vi "SDSU.vi"(8 "error in":errorcluster, 9 "arguments":string, 10 "function":string, 11 "fd in":i32) -> (0 "error out":errorcluster, 1 "result type":string, 2 "str result":string, 3 "fd out":i32)   [LabVIEW 2016]
uses:
  DBSHAND/private/vis/DatabaseHand_Element_Get(bool).vi
  DBSHAND/private/vis/DatabaseHand_Element_Set(bool).vi
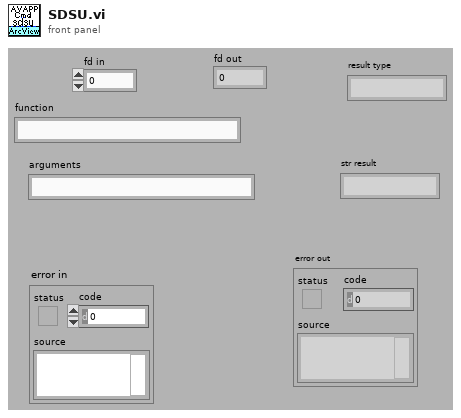
[diagram p1: front panel]
types:
  T1 = cluster{"Video Processor Type":string, "support gain":bool, "Timing Board":string, "support reset":bool, "Utility Board":string, "Shutter":string, "Temperature":string, "support temp control":bool, "Detector Type":string, "Support MPP":string, "Support Binning":string, "Readout Mode":string, "support shutter control":bool}
  T2 = typedef "DatabaseHand_RefNum.ctl" = refnum<vi>
  T3 = typedef "CMN_ContStatus.ctl" = cluster{"Response":string, "power":bool, "shutter":bool, "artifdata":bool, "idlemode":bool, "reset":bool, "gain":u8, "speed":u8, "resetPCI":bool, "autoshutter":bool, "TempSetPoint":i32, "multipleextensions":bool, "displayImage":bool, "coadding":bool, "images being coadded":i32, "Operation Mode":enum16{"normal", "coadd", "fawler"}, "frames to write":cluster{"subs":bool, "reset":bool, "exposed":bool}, "fawler samples":i32, "write auto":bool, "datatype":string, "frames to display":cluster{"subs":bool, "reset":bool, "exposed":bool}, "sur":i32, "autoclear":bool}
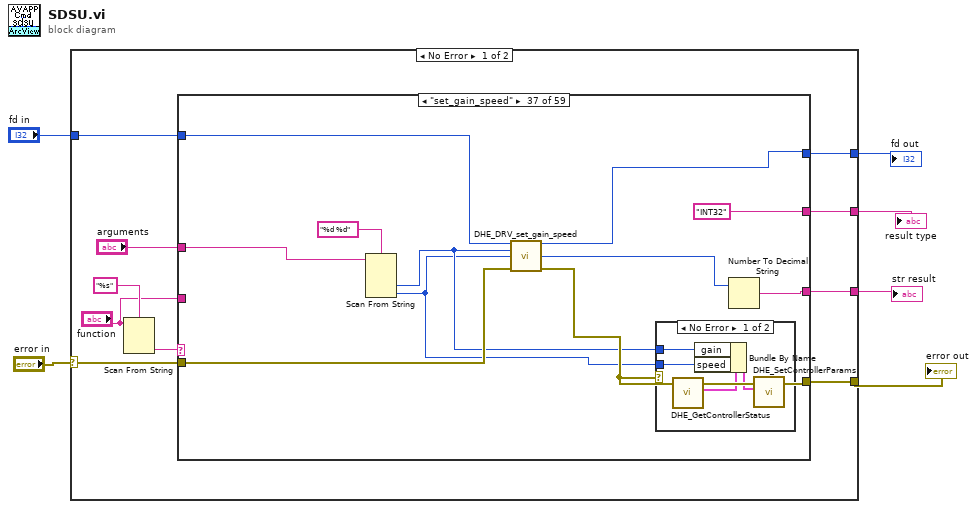
[diagram p0: block diagram]
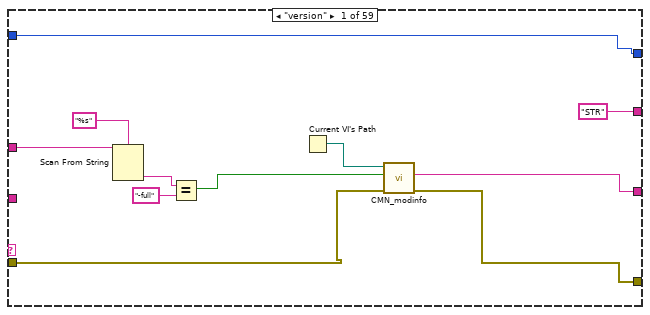
[diagram p2: hidden frame]
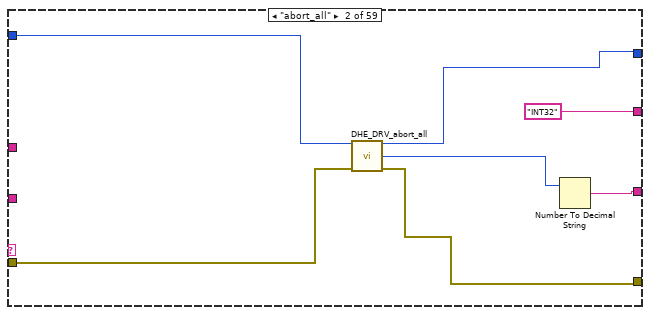
[diagram p3: hidden frame]
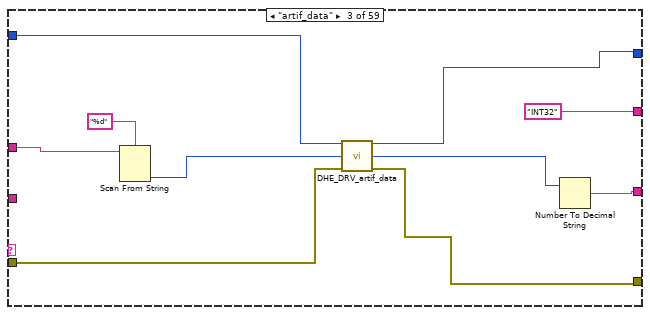
[diagram p4: hidden frame]
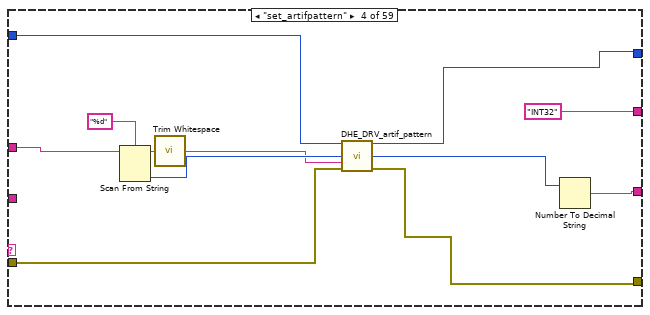
[diagram p5: hidden frame]
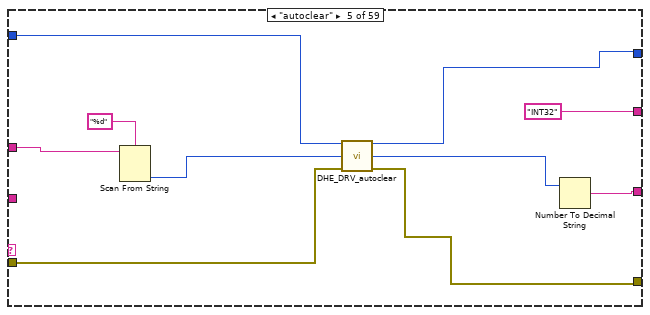
[diagram p6: hidden frame]
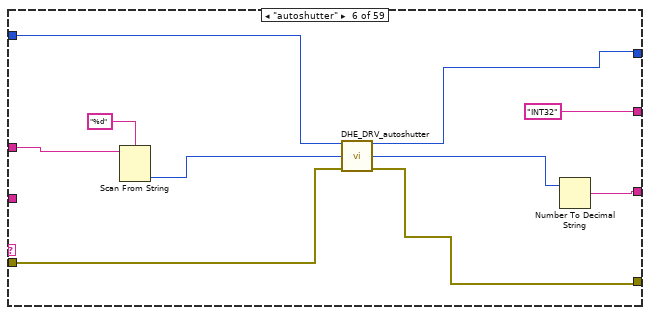
[diagram p7: hidden frame]
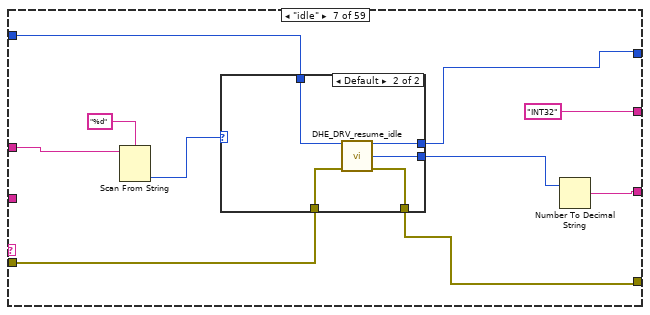
[diagram p8: hidden frame]
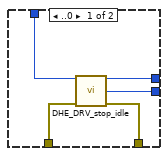
[diagram p9: hidden frame]
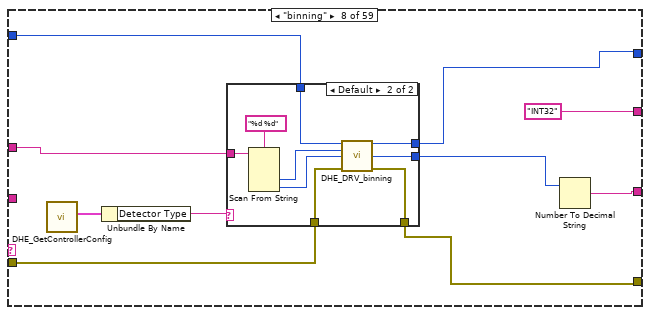
[diagram p10: hidden frame]
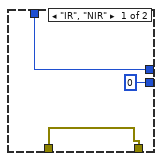
[diagram p11: hidden frame]
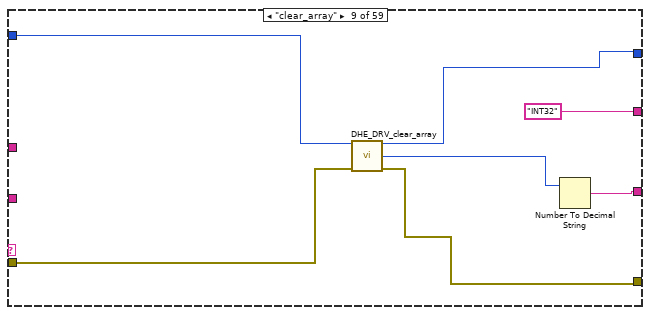
[diagram p12: hidden frame]
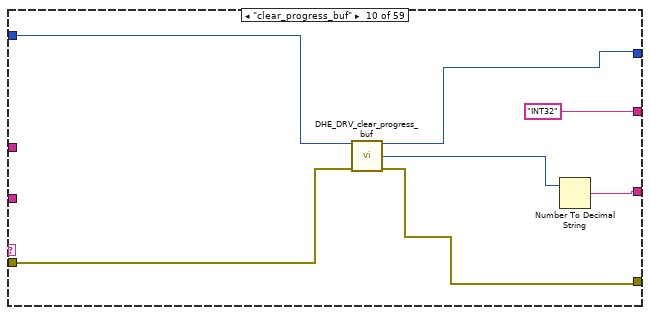
[diagram p13: hidden frame]
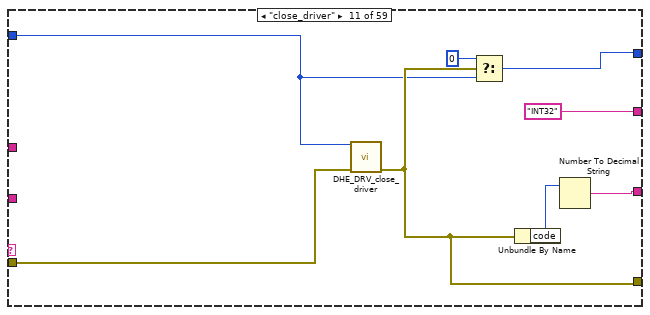
[diagram p14: hidden frame]
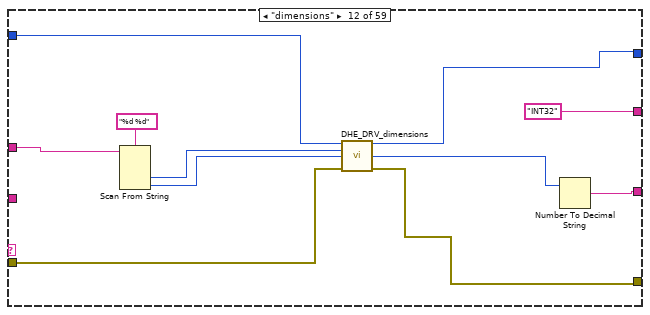
[diagram p15: hidden frame]
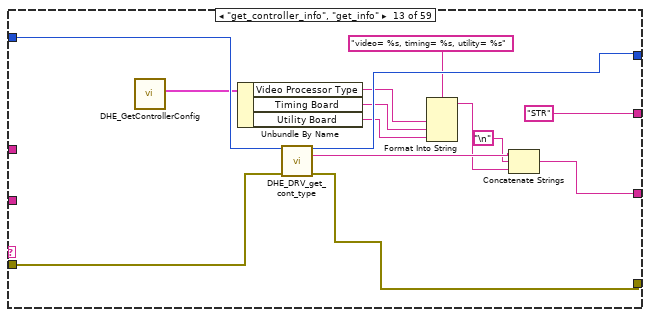
[diagram p16: hidden frame]
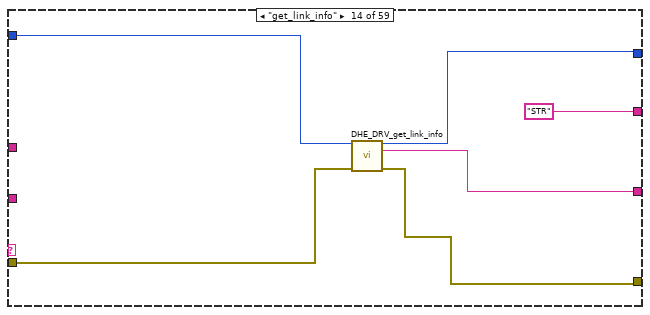
[diagram p17: hidden frame]
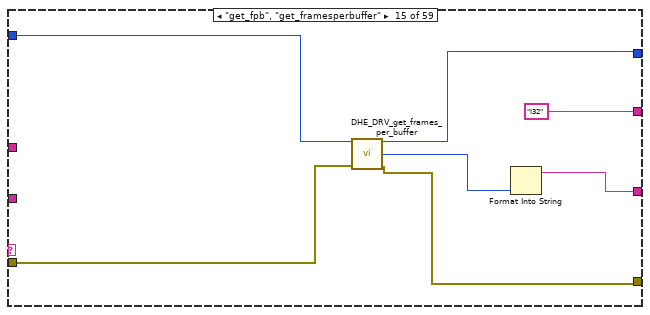
[diagram p18: hidden frame]
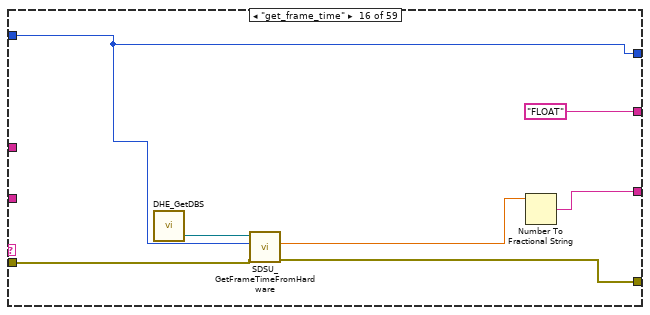
[diagram p19: hidden frame]
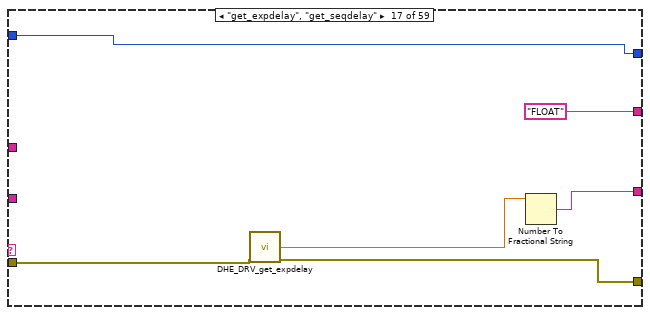
[diagram p20: hidden frame]
diagram:
  n1 = case shown="No Error" "error in" {
    selector: "error in" -> [w10 w645]
    tunnel: [w11 w645] -> w6
    tunnel: [w15 w644] -> w4
    tunnel: "fd in" -> [w14 w644]
    tunnel: [w13 w643] -> w2
    tunnel: [w12 w643] -> w1
    frame No Error {
      n2 = Scan From String(format string="%s", input string="function") -> (output 1=w8:string)  [unwired: 2 in, 4 out]
      n3 = case shown="\"set_gain_speed\"" w8 {
        tunnel: w10 -> [w18 w31 w42 w54 w64 w74 w84 w104 w122 w129 w139 w149 w163 w170 w174 w181 w188 w194 w202 w211 w221 w226 w236 w240 w250 w261 w272 w287 w294 w301 w312 w322 w333 w339 w346 w358 w369 w383 w394 w409 w420 w429 w435 w442 w452 w461 w470 w476 w488 w510 w539 w554 w587 w593 w600 w609 w619 w625 w639]
        tunnel: "arguments" -> [w23 _ w37 w49 w59 w69 w79 w99 _ _ _ w144 _ _ _ _ _ _ _ _ _ _ w231 w246 _ w256 w270 w283 _ _ w307 w317 w329 _ _ w354 w366 w378 w389 w404 w415 w426 _ _ w454 w463 w472 w484 w496 w511 w535 w553 w582 _ _ w605 w621 w629 w636]
        tunnel: [w24 w28 w39 w51 w61 w71 w81 w101 w119 w126 w134 w146 w161 w167 w176 w182 w189 w195 w203 w212 w222 w228 w233 w243 w247 w258 w274 w289 w291 w298 w309 w319 w331 w336 w344 w356 w368 w380 w391 w406 w417 w424 w432 w439 w449 w459 w468 w479 w493 w509 w536 w556 w584 w590 w599 w606 w615 w626 w640] -> w15
        tunnel: w14 -> [w24 w32 w40 w52 w62 w72 w82 w102 w123 w130 w135 w147 w164 w168 w177 w182 w189 w195 w203 w212 w222 w228 w234 _ w251 w259 w275 w290 w295 w302 w310 w320 w327 w340 w347 w352 w364 w381 w392 w407 w418 w424 w432 w440 w450 w459 w468 w480 w494 w509 w540 w557 w585 w594 w599 w607 w616 w627 w641]
        tunnel: [w26 w33 w43 w55 w65 w75 w85 w105 w124 w131 w137 w150 w152 w166 w173 w184 w190 w196 w204 w207 w216 w223 w237 w242 w252 w262 w271 w286 w296 w303 w313 w323 w334 w341 w348 w359 w370 w384 w395 w410 w421 w430 w436 w443 w455 w464 w473 w485 w497 w512 w541 w544 w588 w595 w601 w604 w617 w623 w637] -> w13
        tunnel: ["STR" "INT32" "INT32" "INT32" "INT32" "INT32" "INT32" "INT32" "INT32" "INT32" "INT32" "INT32" "STR" "STR" "I32" "FLOAT" "FLOAT" "FLOAT" "FLOAT" "STR" "STR" "STR" "INT32" "INT32" "INT32" "INT32" "STR" "STR" "INT32" "INT32" "INT32" "INT32" "INT32" "INT32" "INT32" "INT32" "INT32" "INT32" "INT32" "INT32" "INT32" "INT32" "INT32" "FLOAT" "INT32" "INT32" "INT32" "INT32" "INT32" "INT32" "INT32" "INT32" "INT32" "INT32" "INT32" "STR" "STR" "STR" "STR"] -> w12
        tunnel: [w17 w30 w41 w53 w63 w73 w83 w103 w121 w128 w136 w148 w162 w169 w175 w180 w187 w193 w201 w211 w221 w225 w235 w239 w249 w260 w273 w288 w293 w300 w311 w321 w332 w338 w345 w357 w363 w382 w393 w408 w419 w428 w434 w441 w451 w460 w469 w475 w487 w503 w538 w555 w586 w592 w598 w608 w618 w624 w638] -> w11
        tunnel: "function" -> [_ _ _ _ _ _ _ _ _ _ _ _ _ _ _ _ _ _ _ _ _ _ _ _ _ _ _ _ _ _ _ _ _ _ _ _ _ _ _ _ _ _ _ _ _ _ _ _ _ _ _ _ _ _ _ _ _ w631 _]
        frame "version" {
          n4 = Scan From String(format string="%s", input string=w23) -> (output 1=w21:string)  [unwired: 2 in, 4 out]
          n5 = Equal?(x=w21, y="-full") -> (x = y?=w19:bool)
          n6 = Current VI's Path() -> (path=w27:path)
          n7 = call "CMN_modinfo.vi"("error in (no error)"=w18, "full"=w19, "caller path"=w27) -> ("error out"=w17:errorcluster, "INFO"=w26:string)  [unwired: 7 out]
        }
        frame "abort_all" {
          n8 = call "DHE_DRV_abort_all.vi"("fd"=w32, "error in (no error)"=w31) -> ("fd out"=w28:i32, "return value"=w29:i32, "error out"=w30:errorcluster)  [unwired: 11 out]
          n9 = Number To Decimal String(number=w29) -> (decimal integer string=w33:string)  [unwired: 1 out]
        }
        frame "artif_data" {
          n10 = Scan From String(format string="%d", input string=w37) -> (output 1=w35:i32)  [unwired: 2 in, 4 out]
          n11 = call "DHE_DRV_artif_data.vi"("fd"=w40, "flag"=w35, "error in (no error)"=w42) -> ("fd out"=w39:i32, "return value"=w38:i32, "error out"=w41:errorcluster)  [unwired: 10 out]
          n12 = Number To Decimal String(number=w38) -> (decimal integer string=w43:string)  [unwired: 1 out]
        }
        frame "set_artifpattern" {
          n13 = Scan From String(format string="%d", input string=w49) -> (remaining string=w46:string, output 1=w47:i32)  [unwired: 2 in, 3 out]
          n14 = call <vilib>:"Trim Whitespace.vi"("string"=w46) -> ("trimmed string"=w45:string)  [unwired: 1 in]
          n15 = call "DHE_DRV_artif_pattern.vi"("fd"=w52, "type"=w47, "params"=w45, "error in (no error)"=w54) -> ("fd out"=w51:i32, "return value"=w50:i32, "error out"=w53:errorcluster)  [unwired: 9 out]
          n16 = Number To Decimal String(number=w50) -> (decimal integer string=w55:string)  [unwired: 1 out]
        }
        frame "autoclear" {
          n17 = Scan From String(format string="%d", input string=w59) -> (output 1=w57:i32)  [unwired: 2 in, 4 out]
          n18 = call "DHE_DRV_autoclear.vi"("fd"=w62, "flag"=w57, "error in (no error)"=w64) -> ("fd out"=w61:i32, "return value"=w60:i32, "error out"=w63:errorcluster)  [unwired: 10 out]
          n19 = Number To Decimal String(number=w60) -> (decimal integer string=w65:string)  [unwired: 1 out]
        }
        frame "autoshutter" {
          n20 = Scan From String(format string="%d", input string=w69) -> (output 1=w67:i32)  [unwired: 2 in, 4 out]
          n21 = call "DHE_DRV_autoshutter.vi"("fd"=w72, "flag"=w67, "error in (no error)"=w74) -> ("fd out"=w71:i32, "return value"=w70:i32, "error out"=w73:errorcluster)  [unwired: 10 out]
          n22 = Number To Decimal String(number=w70) -> (decimal integer string=w75:string)  [unwired: 1 out]
        }
        frame "idle" {
          n23 = Scan From String(format string="%d", input string=w79) -> (output 1=w77:i32)  [unwired: 2 in, 4 out]
          n24 = case shown="Default" w77 {
            tunnel: w84 -> [w91 w96]
            tunnel: [w90 w95] -> w83
            tunnel: w82 -> [w89 w94]
            tunnel: [w88 w93] -> w81
            tunnel: [w87 w92] -> w80
            frame ..0 {
              n25 = call "DHE_DRV_stop_idle.vi"("fd"=w89, "error in (no error)"=w91) -> ("fd out"=w88:i32, "return value"=w87:i32, "error out"=w90:errorcluster)  [unwired: 11 out]
            }
            frame Default {
              n26 = call "DHE_DRV_resume_idle.vi"("fd"=w94, "error in (no error)"=w96) -> ("fd out"=w93:i32, "return value"=w92:i32, "error out"=w95:errorcluster)  [unwired: 11 out]
            }
          }
          n27 = Number To Decimal String(number=w80) -> (decimal integer string=w85:string)  [unwired: 1 out]
        }
        frame "binning" {
          n28 = call "DHE_GetControllerConfig.vi"() -> ("ControllerConfigCluster"=w98:T1)  [unwired: 11 out]
          n29 = Unbundle By Name(w98) -> ("Detector Type"=w97:string)
          n30 = case shown="Default" w97 {
            tunnel: w104 -> [w107 w118]
            tunnel: [w107 w117] -> w103
            tunnel: w102 -> [w109 w116]
            tunnel: [w109 w115] -> w101
            tunnel: [0 ("return value") w114] -> w100
            tunnel: w99 -> [_ w113]
            frame "IR", "NIR" {
            }
            frame Default {
              n31 = Scan From String(format string="%d %d", input string=w113) -> (output 1=w111:i32, output 2=w110:i32)  [unwired: 2 in, 5 out]
              n32 = call "DHE_DRV_binning.vi"("fd"=w116, "xbin"=w111, "ybin"=w110, "error in (no error)"=w118) -> ("fd out"=w115:i32, "return value"=w114:i32, "error out"=w117:errorcluster)  [unwired: 9 out]
            }
          }
          n33 = Number To Decimal String(number=w100) -> (decimal integer string=w105:string)  [unwired: 1 out]
        }
        frame "clear_array" {
          n34 = call "DHE_DRV_clear_array.vi"("fd"=w123, "error in (no error)"=w122) -> ("fd out"=w119:i32, "return value"=w120:i32, "error out"=w121:errorcluster)  [unwired: 11 out]
          n35 = Number To Decimal String(number=w120) -> (decimal integer string=w124:string)  [unwired: 1 out]
        }
        frame "clear_progress_buf" {
          n36 = call "DHE_DRV_clear_progress_buf.vi"("fd"=w130, "error in (no error)"=w129) -> ("fd"=w126:i32, "return value"=w127:i32, "error out"=w128:errorcluster)  [unwired: 11 out]
          n37 = Number To Decimal String(number=w127) -> (decimal integer string=w131:string)  [unwired: 1 out]
        }
        frame "close_driver" {
          n38 = call "DHE_DRV_close_driver.vi"("fd"=w135, "error in (no error)"=w139) -> ("error out"=w136:errorcluster)  [unwired: 13 out]
          n39 = Select(t=0, s=w136, f=w135) -> (s? t:f=w134:i32)
          n40 = Unbundle By Name(w136) -> ("code"=w138:i32)
          n41 = Number To Decimal String(number=w138) -> (decimal integer string=w137:string)  [unwired: 1 out]
        }
        frame "dimensions" {
          n42 = Scan From String(format string="%d %d", input string=w144) -> (output 1=w142:i32, output 2=w141:i32)  [unwired: 2 in, 5 out]
          n43 = call "DHE_DRV_dimensions.vi"("fd"=w147, "Columns"=w142, "Rows"=w141, "error in (no error)"=w149) -> ("fd out"=w146:i32, "return value"=w145:i32, "error out"=w148:errorcluster)  [unwired: 9 out]
          n44 = Number To Decimal String(number=w145) -> (decimal integer string=w150:string)  [unwired: 1 out]
        }
        frame "get_controller_info", "get_info" {
          n45 = call "DHE_GetControllerConfig.vi"() -> ("ControllerConfigCluster"=w160:T1)  [unwired: 11 out]
          n46 = Unbundle By Name(w160) -> ("Video Processor Type"=w157:string, "Timing Board"=w156:string, "Utility Board"=w155:string)
          n47 = call "DHE_DRV_get_cont_type.vi"("fd"=w164, "error in (no error)"=w163) -> ("fd out"=w161:i32, "info out"=w159:string, "error out"=w162:errorcluster)  [unwired: 11 out]
          n48 = Format Into String(format string="video= %s, timing= %s, utility= %s", w157, w156, w155) -> (resulting string=w153:string)  [unwired: 2 in, 1 out]
          n49 = Concatenate Strings(w159, "\n", w153) -> (w152:string)
        }
        frame "get_link_info" {
          n50 = call "DHE_DRV_get_link_info.vi"("fd"=w168, "error in (no error)"=w170) -> ("fd out"=w167:i32, "info out"=w166:string, "error out"=w169:errorcluster)  [unwired: 11 out]
        }
        frame "get_fpb", "get_framesperbuffer" {
          n51 = call "DHE_DRV_get_frames_per_buffer.vi"("fd"=w177, "error in (no error)"=w174) -> ("fd"=w176:i32, "fpb"=w172:i32, "error out"=w175:errorcluster)  [unwired: 11 out]
          n52 = Format Into String(w172) -> (resulting string=w173:string)  [unwired: 3 in, 1 out]
        }
        frame "get_frame_time" {
          n53 = call "DHE_GetDBS.vi"() -> ("DHE_DBSRef"=w183:T2)  [unwired: 9 out]
          n54 = call "SDSU_GetFrameTimeFromHardware.vi"("error in"=w181, "fd"=w182, "Database Ref"=w183) -> ("errorout"=w180:errorcluster, "frame_time"=w179:dbl)  [unwired: 7 out]
          n55 = Number To Fractional String(number=w179) -> (F-format string=w184:string)  [unwired: 3 out]
        }
        frame "get_expdelay", "get_seqdelay" {
          n56 = call "DHE_DRV_get_expdelay.vi"("error in (no error)"=w188) -> ("delay"=w186:sgl, "error out"=w187:errorcluster)  [unwired: 2 in, 11 out]
          n57 = Number To Fractional String(number=w186) -> (F-format string=w190:string)  [unwired: 3 out]
        }
        frame "get_iniexpdelay", "get_iniseqdelay", "get_initdelay", "get_intdelay" {
          n58 = call "DHE_DRV_get_iniexpdelay.vi"("error in (no error)"=w194) -> ("delay"=w192:sgl, "error out"=w193:errorcluster)  [unwired: 13 out]
          n59 = Number To Fractional String(number=w192) -> (F-format string=w196:string)  [unwired: 3 out]
        }
        frame "get_act_inttime", "get_actual_inttime", "get_hard_inttime" {
          n60 = call "DHE_DRV_get_actual_inttime.vi"("error in (no error)"=w202) -> ("actual inttime"=w200:i32, "error out"=w201:errorcluster)  [unwired: 13 out]
          n61 = Divide(x=w200, y=1000) -> (x/y=w198:dbl)
          n62 = Number To Fractional String(number=w198) -> (F-format string=w204:string)  [unwired: 3 out]
        }
        frame "get_samplings" {
          n63 = call "DHE_GetControllerConfig.vi"() -> ("ControllerConfigCluster"=w210:T1)  [unwired: 11 out]
          n64 = Unbundle By Name(w210) -> ("Detector Type"=w209:string)
          n65 = To Lower Case(string=w209) -> (all lower case string=w208:string)
          n66 = case shown="Default" w208 {
            tunnel: ["single, singframe" "single, cds, fowler, sur"] -> w207
            frame Default {
            }
            frame "ir", "nir" {
            }
          }
        }
        frame "get_sync" {
          n67 = call "DHE_GetDBS.vi"() -> ("DHE_DBSRef"=w215:T2)  [unwired: 9 out]
          n68 = call-poly "DatabaseHand_Get.vi"("default value"=FALSE, "name"="synced", "Database RefNum in"=w215) -> ("value"=w217:bool)  [unwired: 2 in, 6 out]
          n69 = Format Into String(w217) -> (resulting string=w216:string)  [unwired: 3 in, 1 out]
        }
        frame "get_guide_mode" {
          n70 = call "DHE_DRV_get_guide_mode.vi"("error in (no error)"=w226) -> ("guide_mode"=w224:bool, "error out"=w225:errorcluster)  [unwired: 13 out]
          n71 = Format Into String(w224) -> (resulting string=w223:string)  [unwired: 3 in, 1 out]
        }
        frame "move_shutter" {
          n72 = Scan From String(format string="%d", input string=w231) -> (output 1=w229:i32)  [unwired: 2 in, 4 out]
          n73 = call "DHE_DRV_move_shutter.vi"("fd"=w234, "flag"=w229, "error in (no error)"=w236) -> ("fd out"=w233:i32, "return value"=w232:i32, "error out"=w235:errorcluster)  [unwired: 10 out]
          n74 = Number To Decimal String(number=w232) -> (decimal integer string=w237:string)  [unwired: 1 out]
        }
        frame "open_driver" {
          n75 = Scan From String(format string="%d", input string=w246) -> (output 1=w244:i32)  [unwired: 2 in, 4 out]
          n76 = call "DHE_DRV_open_driver.vi"("devno"=w244, "error in (no error)"=w240) -> ("refnum"=w243:i32, "error out"=w239:errorcluster)  [unwired: 12 out]
          n77 = Format Into String(w243) -> (resulting string=w242:string)  [unwired: 3 in, 1 out]
        }
        frame "pause_exposure" {
          n78 = call "DHE_DRV_pause_exposure.vi"("fd"=w251, "error in (no error)"=w250) -> ("fd out"=w247:i32, "return value"=w248:i32, "error out"=w249:errorcluster)  [unwired: 11 out]
          n79 = Number To Decimal String(number=w248) -> (decimal integer string=w252:string)  [unwired: 1 out]
        }
        frame "power" {
          n80 = Scan From String(format string="%d", input string=w256) -> (output 1=w254:i32)  [unwired: 2 in, 4 out]
          n81 = call "DHE_DRV_power.vi"("fd"=w259, "flag"=w254, "error in (no error)"=w261) -> ("fd out"=w258:i32, "return value"=w257:i32, "error out"=w260:errorcluster)  [unwired: 10 out]
          n82 = Number To Decimal String(number=w257) -> (decimal integer string=w262:string)  [unwired: 1 out]
        }
        frame "read_memory", "read_temperature", "read_tp" {
          # "board memory address"
          n83 = Scan From String(format string="%s %s %s", input string=w270) -> (output 1=w268:string, output 2=w267:string, output 3=w266:string)  [unwired: 2 in, 6 out]
          n84 = Format Into String(format string="read %s %s %s " ("string"), w268, w267, w266) -> (resulting string=w265:string)  [unwired: 2 in, 1 out]
          n85 = call "SDSU_Memory.vi"("refnum"=w275, "Command In"=w265, "error in (no error)"=w272) -> ("refnum out"=w274:i32, "message"=w271:string, "error out"=w273:errorcluster)  [unwired: 2 in, 8 out]
        }
        frame "write_memory", "write_tp" {
          # "board memory address type value name"
          # "board memory address value"
          n86 = Scan From String(format string="%s %s %s %s %s %s ", input string=w283) -> (output 1=w284:string, output 2=w282:string, output 3=w281:string, output 5=w279:string)  [unwired: 2 in, 11 out]
          n87 = Format Into String(format string="write %s %s %s %s " ("string"), w284, w282, w281, w279) -> (resulting string=w277:string)  [unwired: 2 in, 1 out]
          n88 = call "SDSU_Memory.vi"("refnum"=w290, "Command In"=w277, "error in (no error)"=w287) -> ("refnum out"=w289:i32, "message"=w286:string, "error out"=w288:errorcluster)  [unwired: 2 in, 8 out]
        }
        frame "reset_controller" {
          n89 = call "DRV_SDSU_reset_ctrler.vi"("fd"=w295, "error in (no error)"=w294) -> ("fd out"=w291:i32, "return value"=w292:i32, "error out"=w293:errorcluster)  [unwired: 11 out]
          n90 = Number To Decimal String(number=w292) -> (decimal integer string=w296:string)  [unwired: 1 out]
        }
        frame "resume_exposure" {
          n91 = call "DHE_DRV_resume_exposure.vi"("fd"=w302, "error in (no error)"=w301) -> ("fd out"=w298:i32, "return value"=w299:i32, "error out"=w300:errorcluster)  [unwired: 11 out]
          n92 = Number To Decimal String(number=w299) -> (decimal integer string=w303:string)  [unwired: 1 out]
        }
        frame "set_bpp" {
          n93 = Scan From String(format string="%d", input string=w307) -> (output 1=w305:i32)  [unwired: 2 in, 4 out]
          n94 = call "DHE_DRV_set_bpp.vi"("fd"=w310, "bpp"=w305, "error in (no error)"=w312) -> ("fd out"=w309:i32, "return value"=w308:i32, "error out"=w311:errorcluster)  [unwired: 10 out]
          n95 = Number To Decimal String(number=w308) -> (decimal integer string=w313:string)  [unwired: 1 out]
        }
        frame "set_pixel_time", "set_pixeltime", "set_pixtime" {
          n96 = Scan From String(format string="%g", input string=w317) -> (output 1=w315:dbl)  [unwired: 2 in, 4 out]
          n97 = call "DHE_DRV_set_pixeltime.vi"("fd"=w320, "pixtime"=w315, "error in (no error)"=w322) -> ("fd out"=w319:i32, "return value"=w318:i32, "error out"=w321:errorcluster)  [unwired: 10 out]
          n98 = Number To Decimal String(number=w318) -> (decimal integer string=w323:string)  [unwired: 1 out]
        }
        frame "set_gain" {
          n99 = call "DHE_DRV_get_gain_speed.vi"("fd"=w327) -> ("speed"=w325:i32)  [unwired: 10 in, 4 out]
          n100 = Scan From String(format string="%d", input string=w329) -> (output 1=w326:i32)  [unwired: 2 in, 4 out]
          n101 = call "DHE_DRV_set_gain_speed.vi"("fd"=w327, "gain"=w326, "speed"=w325, "error in (no error)"=w333) -> ("fd out"=w331:i32, "return value"=w330:i32, "error out"=w332:errorcluster)  [unwired: 9 in]
          n102 = Number To Decimal String(number=w330) -> (decimal integer string=w334:string)  [unwired: 1 out]
        }
        frame "get_gain" {
          n103 = call "DHE_DRV_get_gain_speed.vi"("fd"=w340, "error in (no error)"=w339) -> ("fd out"=w336:i32, "gain"=w337:i32, "error out"=w338:errorcluster)  [unwired: 9 in, 2 out]
          n104 = Number To Decimal String(number=w337) -> (decimal integer string=w341:string)  [unwired: 1 out]
        }
        frame "get_speed" {
          n105 = call "DHE_DRV_get_gain_speed.vi"("fd"=w347, "error in (no error)"=w346) -> ("fd out"=w344:i32, "speed"=w343:i32, "error out"=w345:errorcluster)  [unwired: 9 in, 2 out]
          n106 = Number To Decimal String(number=w343) -> (decimal integer string=w348:string)  [unwired: 1 out]
        }
        frame "set_speed" {
          n107 = call "DHE_DRV_get_gain_speed.vi"("fd"=w352) -> ("gain"=w351:i32)  [unwired: 10 in, 4 out]
          n108 = Scan From String(format string="%d", input string=w354) -> (output 1=w350:i32)  [unwired: 2 in, 4 out]
          n109 = call "DHE_DRV_set_gain_speed.vi"("fd"=w352, "gain"=w351, "speed"=w350, "error in (no error)"=w358) -> ("fd out"=w356:i32, "return value"=w355:i32, "error out"=w357:errorcluster)  [unwired: 9 in]
          n110 = Number To Decimal String(number=w355) -> (decimal integer string=w359:string)  [unwired: 1 out]
        }
        frame "set_gain_speed" {
          n111 = Scan From String(format string="%d %d", input string=w366) -> (output 1=w362:i32, output 2=w361:i32)  [unwired: 2 in, 5 out]
          n112 = call "DHE_DRV_set_gain_speed.vi"("fd"=w364, "gain"=w362, "speed"=w361, "error in (no error)"=w369) -> ("fd out"=w368:i32, "return value"=w367:i32, "error out"=w363:errorcluster)  [unwired: 9 in]
          n113 = case shown="No Error" w363 {
            tunnel: w362 -> [w373 _]
            tunnel: w361 -> [w372 _]
            frame No Error {
              n114 = call "DHE_GetControllerStatus.vi"() -> ("ControllerStatus"=w375:T3)  [unwired: 11 out]
              n115 = Bundle By Name(cluster=w375, "gain"=w373, "speed"=w372) -> (w374:T3)
              n116 = call "DHE_SetControllerParams.vi"("ControllerStatus"=w374) -> ()  [unwired: 1 in, 10 out]
            }
            frame Error {
            }
          }
          n117 = Number To Decimal String(number=w367) -> (decimal integer string=w370:string)  [unwired: 1 out]
        }
        frame "framesperbuffer", "set_fpb", "set_framesperbuffer" {
          n118 = Scan From String(format string="%d", input string=w378) -> (output 1=w376:i32)  [unwired: 2 in, 4 out]
          n119 = call "DHE_DRV_set_fpb.vi"("fd"=w381, "fpb"=w376, "error in (no error)"=w383) -> ("fd out"=w380:i32, "return value"=w379:i32, "error out"=w382:errorcluster)  [unwired: 10 out]
          n120 = Number To Decimal String(number=w379) -> (decimal integer string=w384:string)  [unwired: 1 out]
        }
        frame "set_exp_time" {
          n121 = Scan From String(format string="%d", input string=w389) -> (output 1=w387:i32)  [unwired: 2 in, 4 out]
          n122 = To Unsigned Long Integer(number=w387) -> (unsigned 32bit integer=w386:u32)
          n123 = call "DHE_DRV_set_exp_time.vi"("fd"=w392, "val"=w386, "error in (no error)"=w394) -> ("fd out"=w391:i32, "return value"=w390:i32, "error out"=w393:errorcluster)  [unwired: 10 out]
          n124 = Number To Decimal String(number=w390) -> (decimal integer string=w395:string)  [unwired: 1 out]
        }
        frame "set_geom" {
          # "xpre xdata xpost ypre ydata ypost"
          n125 = Scan From String(format string="%d %d %d %d %d %d", input string=w404) -> (output 1=w402:i32, output 2=w401:i32, output 3=w400:i32, output 4=w398:i32, output 5=w399:i32, output 6=w397:i32)  [unwired: 2 in, 9 out]
          n126 = call "DHE_DRV_set_geom.vi"("fd"=w407, "ypredata"=w398, "ypostdata"=w397, "xpredata"=w402, "xpostdata"=w400, "xdata"=w401, "error in (no error)"=w409, "ydata"=w399) -> ("fd out"=w406:i32, "return value"=w405:i32, "error out"=w408:errorcluster)  [unwired: 5 out]
          n127 = Number To Decimal String(number=w405) -> (decimal integer string=w410:string)  [unwired: 1 out]
        }
        frame "set_nimages" {
          n128 = Scan From String(format string="%d", input string=w415) -> (output 1=w413:i32)  [unwired: 2 in, 4 out]
          n129 = To Unsigned Long Integer(number=w413) -> (unsigned 32bit integer=w412:u32)
          n130 = call "DHE_DRV_set_nimages.vi"("fd"=w418, "nimages"=w412, "error in (no error)"=w420) -> ("fd out"=w417:i32, "return value"=w416:i32, "error out"=w419:errorcluster)  [unwired: 10 out]
          n131 = Number To Decimal String(number=w416) -> (decimal integer string=w421:string)  [unwired: 1 out]
        }
        frame "set_mapping", "set_mapsize" {
          n132 = Scan From String(format string="%d", input string=w426) -> (output 1=w423:i32)  [unwired: 2 in, 4 out]
          n133 = call "DHE_DRV_set_mapsize.vi"("size_MB"=w423, "error in (no error)"=w429) -> ("return value"=w427:i32, "error out"=w428:errorcluster)  [unwired: 2 in, 10 out]
          n134 = Number To Decimal String(number=w427) -> (decimal integer string=w430:string)  [unwired: 1 out]
        }
        frame "get_mapping", "get_mapsize" {
          n135 = call "DHE_DRV_get_mapsize.vi"("error in (no error)"=w435) -> ("return value"=w433:i32, "error out"=w434:errorcluster)  [unwired: 1 in, 12 out]
          n136 = Number To Decimal String(number=w433) -> (decimal integer string=w436:string)  [unwired: 1 out]
        }
        frame "get_pixel_time", "get_pixeltime", "get_pixtime" {
          n137 = call "DHE_DRV_get_pixtime.vi"("fd"=w440, "error in (no error)"=w442) -> ("fd out"=w439:i32, "pixtime"=w438:sgl, "error out"=w441:errorcluster)  [unwired: 11 out]
          n138 = Number To Fractional String(number=w438) -> (F-format string=w443:string)  [unwired: 3 out]
        }
        frame "set_nsur" {
          n139 = Scan From String(format string="%d", input string=w454) -> (output 1=w446:i32)  [unwired: 2 in, 4 out]
          n140 = Max & Min(x=w446, y=1) -> (max(x,y)=w445:i32)  [unwired: 1 out]
          n141 = call "DHE_DRV_set_num_sur.vi"("fd"=w450, "num_reads"=w445, "error in (no error)"=w452) -> ("fd out"=w449:i32, "return value"=w448:i32, "error out"=w451:errorcluster)  [unwired: 10 out]
          n142 = Number To Decimal String(number=w448) -> (decimal integer string=w455:string)  [unwired: 1 out]
        }
        frame "set_expdelay", "set_seqdelay" {
          n143 = Scan From String(format string="%g", input string=w463) -> (output 1=w458:dbl)  [unwired: 2 in, 4 out]
          n144 = call "DHE_DRV_set_expdelay.vi"("delay(ms)"=w458, "error in (no error)"=w461) -> ("error out"=w460:errorcluster)  [unwired: 1 in, 12 out]
          n145 = Number To Decimal String(number=0) -> (decimal integer string=w464:string)  [unwired: 1 out]
        }
        frame "set_inidelay", "set_iniexpdelay", "set_iniseqdelay", "set_intdelay" {
          n146 = Scan From String(format string="%g", input string=w472) -> (output 1=w466:dbl)  [unwired: 2 in, 4 out]
          n147 = call "DHE_DRV_set_iniexpdelay.vi"("delay(ms)"=w466, "error in (no error)"=w470) -> ("error out"=w469:errorcluster)  [unwired: 1 in, 12 out]
          n148 = Number To Decimal String(number=0) -> (decimal integer string=w473:string)  [unwired: 1 out]
        }
        frame "set_ncoadds" {
          n149 = Scan From String(format string="%d", input string=w484) -> (output 1=w481:i32)  [unwired: 2 in, 4 out]
          n150 = Max & Min(x=w481, y=1) -> (max(x,y)=w478:i32)  [unwired: 1 out]
          n151 = call "DHE_DRV_set_num_coadds.vi"("fd"=w480, "num_coadds"=w478, "error in (no error)"=w476) -> ("fd out"=w479:i32, "return value"=w477:i32, "error out"=w475:errorcluster)  [unwired: 10 out]
          n152 = Number To Decimal String(number=w477) -> (decimal integer string=w485:string)  [unwired: 1 out]
        }
        frame "set_fowler", "set_fsamples" {
          n153 = Scan From String(format string="%d", input string=w496) -> (output 1=w491:i32)  [unwired: 2 in, 4 out]
          n154 = Max & Min(x=w491, y=1) -> (max(x,y)=w489:i32)  [unwired: 1 out]
          n155 = call "DHE_DRV_set_num_reads.vi"("fd"=w494, "num_reads"=w489, "error in (no error)"=w488) -> ("fd out"=w493:i32, "return value"=w492:i32, "error out"=w487:errorcluster)  [unwired: 10 out]
          n156 = Number To Decimal String(number=w492) -> (decimal integer string=w497:string)  [unwired: 1 out]
        }
        frame "set_sync" {
          n157 = To Lower Case(string=w511) -> (all lower case string=w501:string)
          n158 = Scan From String(format string="%s", input string=w501) -> (output 1=w499:string)  [unwired: 2 in, 4 out]
          n159 = case shown="\"false\", \"no\", \"off\"" w499 {
            tunnel: w510 -> [w527 w531 w534]
            tunnel: [w523 w531 w534] -> w508
            tunnel: [i16 0 ("flag") i16 1 ("flag") i16 0 ("flag")] -> w506
            tunnel: [FALSE TRUE FALSE] -> w502
            frame Default {
              n160 = Bundle By Name(cluster=w527, "status"=FALSE, "code"=-22, "source"="ERROR <on | off>") -> (w523:errorcluster)
            }
            frame "on", "true", "yes" {
            }
            frame "false", "no", "off" {
            }
          }
          n161 = call "DHE_DRV_sync.vi"("fd"=w509, "flag"=w506, "error in (no error)"=w508) -> ("return value"=w505:i32, "error out"=w507:errorcluster)  [unwired: 11 out]
          n162 = case shown="No Error" w507 {
            selector: w507 -> [w518 w521]
            tunnel: w505 -> [w519 _]
            tunnel: [w519 w520] -> w504
            tunnel: [w518 w521] -> w503
            tunnel: w502 -> [w514 _]
            frame No Error {
              n163 = call "DHE_GetDBS.vi"() -> ("DHE_DBSRef"=w517:T2)  [unwired: 9 out]
              n164 = call-poly "DatabaseHand_Set.vi"("group"="dhe", "name"="synced", "value"=w514, "Database RefNum in"=w517) -> ()  [unwired: 4 in, 4 out]
            }
            frame Error {
              n165 = Unbundle By Name(w521) -> ("code"=w520:i32)
            }
          }
          n166 = Number To Decimal String(number=w504) -> (decimal integer string=w512:string)  [unwired: 1 out]
        }
        frame "set_sampling" {
          n167 = call "SDSU_SetSampling.vi"("error in"=w539, "sampling type"=w535, "fd"=w540) -> ("error out"=w538:errorcluster, "read value"=w537:i32, "fd"=w536:i32)  [unwired: 6 out]
          n168 = Number To Decimal String(number=w537) -> (decimal integer string=w541:string)  [unwired: 1 out]
        }
        frame "set_guide_mode" {
          # "<on | off> exptime cols rows"
          n169 = Scan From String(format string="%s %d %d %d", input string=w553) -> (output 1=w551:string, output 2=w548:i32, output 3=w547:i32, output 4=w546:i32)  [unwired: 2 in, 7 out]
          n170 = case shown="\"0\", \"disable\", \"false\", \"no\", \"off\"" w551 {
            tunnel: [w573 w574 FALSE] -> w549
            tunnel: [w573 w574 TRUE] -> w550
            frame Default {
              w573 = FALSE
            }
            frame "1", "enable", "on", "true", "yes" {
              w574 = TRUE
            }
            frame "0", "disable", "false", "no", "off" {
            }
          }
          n171 = case shown="True" w550 {
            tunnel: w557 -> [w563 w572]
            tunnel: [w563 w571] -> w556
            tunnel: [w561 w570] -> w555
            tunnel: w554 -> [w562 w569]
            tunnel: w549 -> [_ w568]
            tunnel: w548 -> [_ w567]
            tunnel: w547 -> [_ w566]
            tunnel: w546 -> [_ w565]
            tunnel: [w559 w564] -> w543
            frame False {
              w559 = -22 ("code")
              n172 = Bundle By Name(cluster=w562, "status"=TRUE, "code"=w559, "source"="bad argument") -> (w561:errorcluster)
            }
            frame True {
              n173 = call "DHE_DRV_set_guide_mode.vi"("fd"=w572, "exptime"=w567, "guide"=w568, "error in (no error)"=w569, "rows"=w565, "cols"=w566) -> ("fd out"=w571:i32, "return value"=w564:i32, "error out"=w570:errorcluster)  [unwired: 7 out]
            }
          }
          n174 = Number To Decimal String(number=w543) -> (decimal integer string=w544:string)  [unwired: 1 out]
        }
        frame "set_roi" {
          # "xstart ystart xlen ylen"
          n175 = Scan From String(format string="%d %d %d %d", input string=w582) -> (output 1=w580:i32, output 2=w579:i32, output 3=w578:i32, output 4=w577:i32)  [unwired: 2 in, 7 out]
          n176 = call "DHE_DRV_set_roi.vi"("fd"=w585, "xlenght"=w578, "ylenght"=w577, "xstart"=w580, "ystart"=w579, "error in (no error)"=w587) -> ("fd out"=w584:i32, "return value"=w583:i32, "error out"=w586:errorcluster)  [unwired: 7 out]
          n177 = Number To Decimal String(number=w583) -> (decimal integer string=w588:string)  [unwired: 1 out]
        }
        frame "stop_exposure" {
          n178 = call "DHE_DRV_stop_exposure.vi"("fd"=w594, "error in (no error)"=w593) -> ("fd out"=w590:i32, "read val"=w591:i32, "error out"=w592:errorcluster)  [unwired: 11 out]
          n179 = Number To Decimal String(number=w591) -> (decimal integer string=w595:string)  [unwired: 1 out]
        }
        frame "stop_sequence" {
          n180 = call "DHE_DRV_stop_sequence.vi"("error in (no error)"=w600) -> ("error out"=w598:errorcluster)  [unwired: 14 out]
          n181 = Unbundle By Name(w598) -> ("code"=w597:i32)
          n182 = Number To Decimal String(number=w597) -> (decimal integer string=w601:string)  [unwired: 1 out]
        }
        frame "memory" {
          n183 = call "DHE_GetDBS.vi"() -> ("DHE_DBSRef"=w603:T2)  [unwired: 9 out]
          n184 = call "SDSU_Memory.vi"("refnum"=w607, "Database RefNum in"=w603, "Command In"=w605, "error in (no error)"=w609) -> ("refnum out"=w606:i32, "message"=w604:string, "error out"=w608:errorcluster)  [unwired: 1 in, 8 out]
        }
        frame "reg", "register", "registers" {
          n185 = call "CMN_GetPhysUnit.vi"("command in"=w621) -> ("unit"=w613:string, "command out"=w620:string)  [unwired: 9 out]
          n186 = call "CMN_CommandSwitch.vi"("command in"=w620) -> ("swhitches"=w612:string[], "command out"=w614:string, "arguments"=w611:string[])  [unwired: 1 in, 7 out]
          n187 = call "SDSU_REGS.vi"("refnum"=w616, "Command"=w614, "physical unit"=w613, "swhitches"=w612, "error in (no error)"=w619, "switch arguments"=w611) -> ("refnum out"=w615:i32, "response"=w617:string, "error out"=w618:errorcluster)  [unwired: 7 out]
        }
        frame Default {
          n188 = Match Pattern(string=w631, regular expression="_") -> (before substring=w633:string, after substring=w632:string)  [unwired: 3 out]
          n189 = call <vilib>:"Space Constant.vi"() -> ("String"=w630:string)
          n190 = Concatenate Strings(w633, w630, w632, w630, w629) -> (w628:string)
          n191 = call "SDSU_AttHandling.vi"("error IO"=w625, "arguments"=w628, "refnum"=w627) -> ("err out"=w624:errorcluster, "response"=w623:string, "refnum out"=w626:i32)  [unwired: 6 in]
        }
        frame "att", "attribute", "attributes", "atts", "dac", "dacs" {
          n192 = call "SDSU_AttHandling.vi"("error IO"=w639, "arguments"=w636, "refnum"=w641) -> ("err out"=w638:errorcluster, "response"=w637:string, "refnum out"=w640:i32)  [unwired: 6 in]
        }
      }
    }
    frame Error {
      w643 = ""
    }
  }
  "error out" <- w6
  "str result" <- w2
  "result type" <- w1
  "fd out" <- w4
